vi "FinalLabview.vi"() -> ()   [LabVIEW 2021]
panel:
  out "DummyIndicator 5":dbl
  out "Ball Color":dbl
  out "DummyIndicator 3":dbl
  out "Ball Count":dbl
  out "Ball Color 5":string
  out "Ball Color 4":string
  out "Ball Color 3":string
  out "Ball Color 2":string
  out "Ball Color 1":string
  out "Y Coordinate 5":dbl
  out "X Coordinate 5":dbl
  out "Y Coordinate 4":dbl
  out "X Coordinate 4":dbl
  out "Y Coordinate 3":dbl
  out "X Coordinate 3":dbl
  out "Y Coordinate 2":dbl
  out "X Coordinate 2":dbl
  out "2D Picture":picture
  in  "Display History":bool
  in  "Size of Rectangle":i16
  out "Y Coordinate 1":dbl
  out "X Coordinate 1":dbl
  out "Y":dbl
  out "X":dbl
  in  "SendValue8":dbl
  in  "SendValue7":dbl
  in  "SendValue6":dbl
  in  "SendValue5":dbl
  in  "SendValue4":dbl
  in  "SendValue3":dbl
  in  "SendValue2":dbl
  in  "SendValue1":dbl
  in  "Send Button":bool
  in  "Stop Button":bool
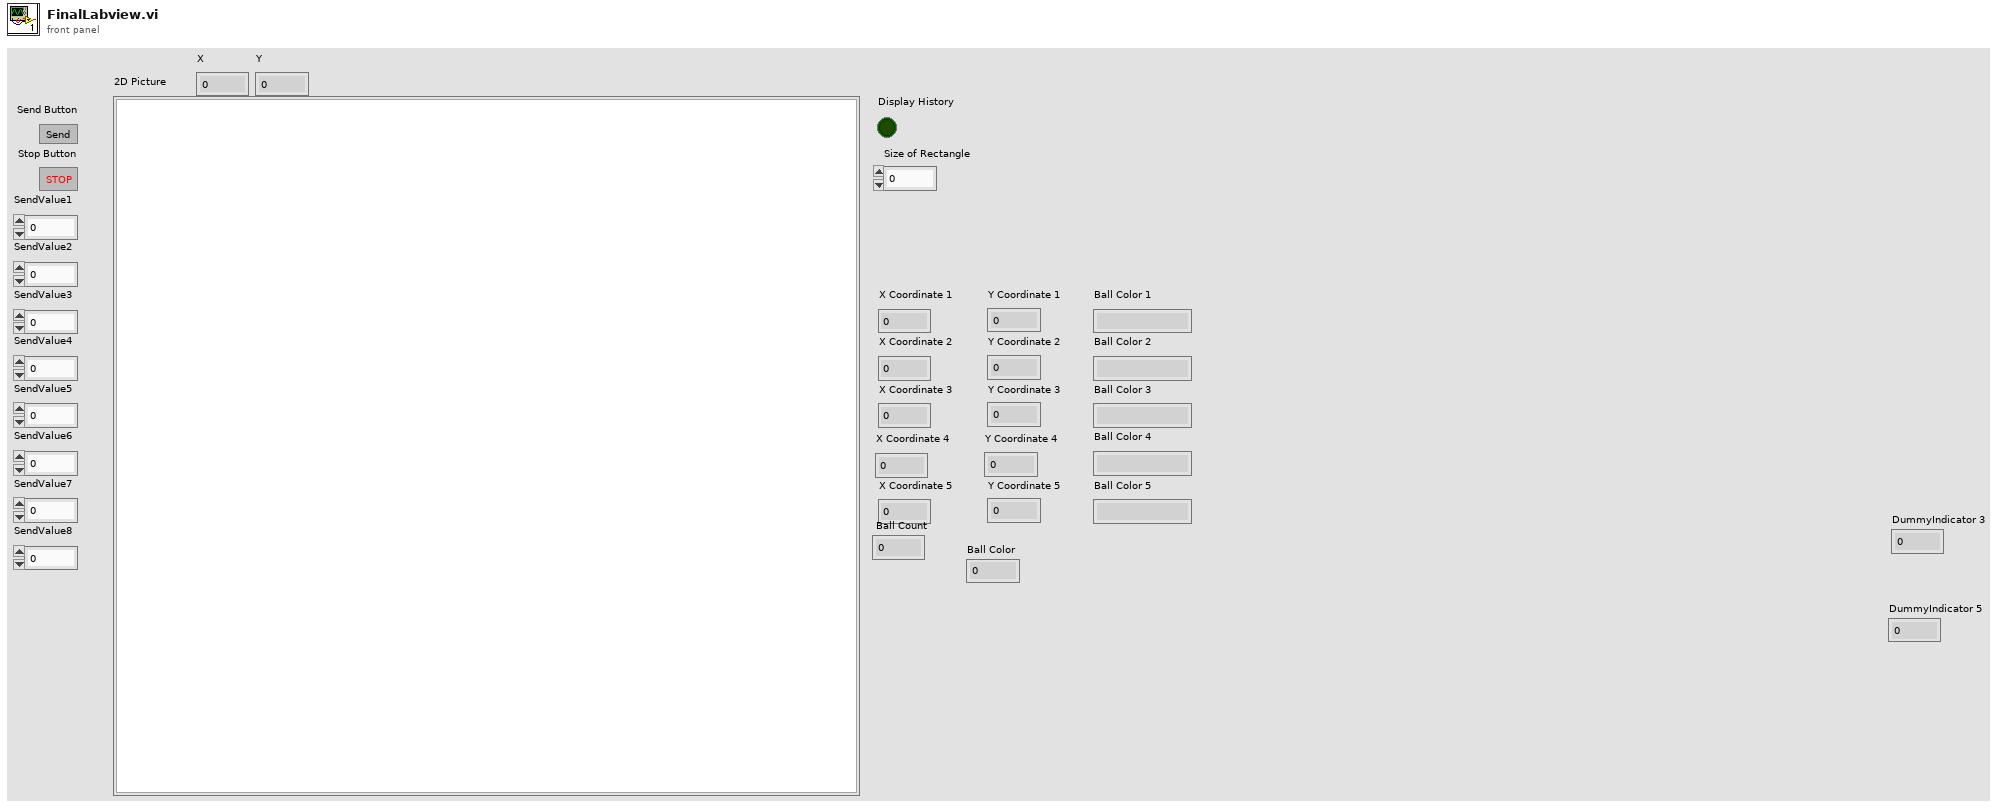
[diagram p1: front panel]
types:
  T1 = cluster{"Width":u16, "Style":enum32{"Solid", "Dash", "Dot", "DashDot", "DashDotDot"}}
  T2 = cluster{"Width":i16, "Style":enum32{"Solid", "Dash", "Dot", "DashDot", "DashDotDot"}}
  T3 = cluster{"left":i16, "top":i16, "right":i16, "bottom":i16}
  T4 = enum16{"Standard", "Buffered", "CRLF", "Immediate"}
  T5 = cluster{"default value 1":dbl, "default value 1":dbl}
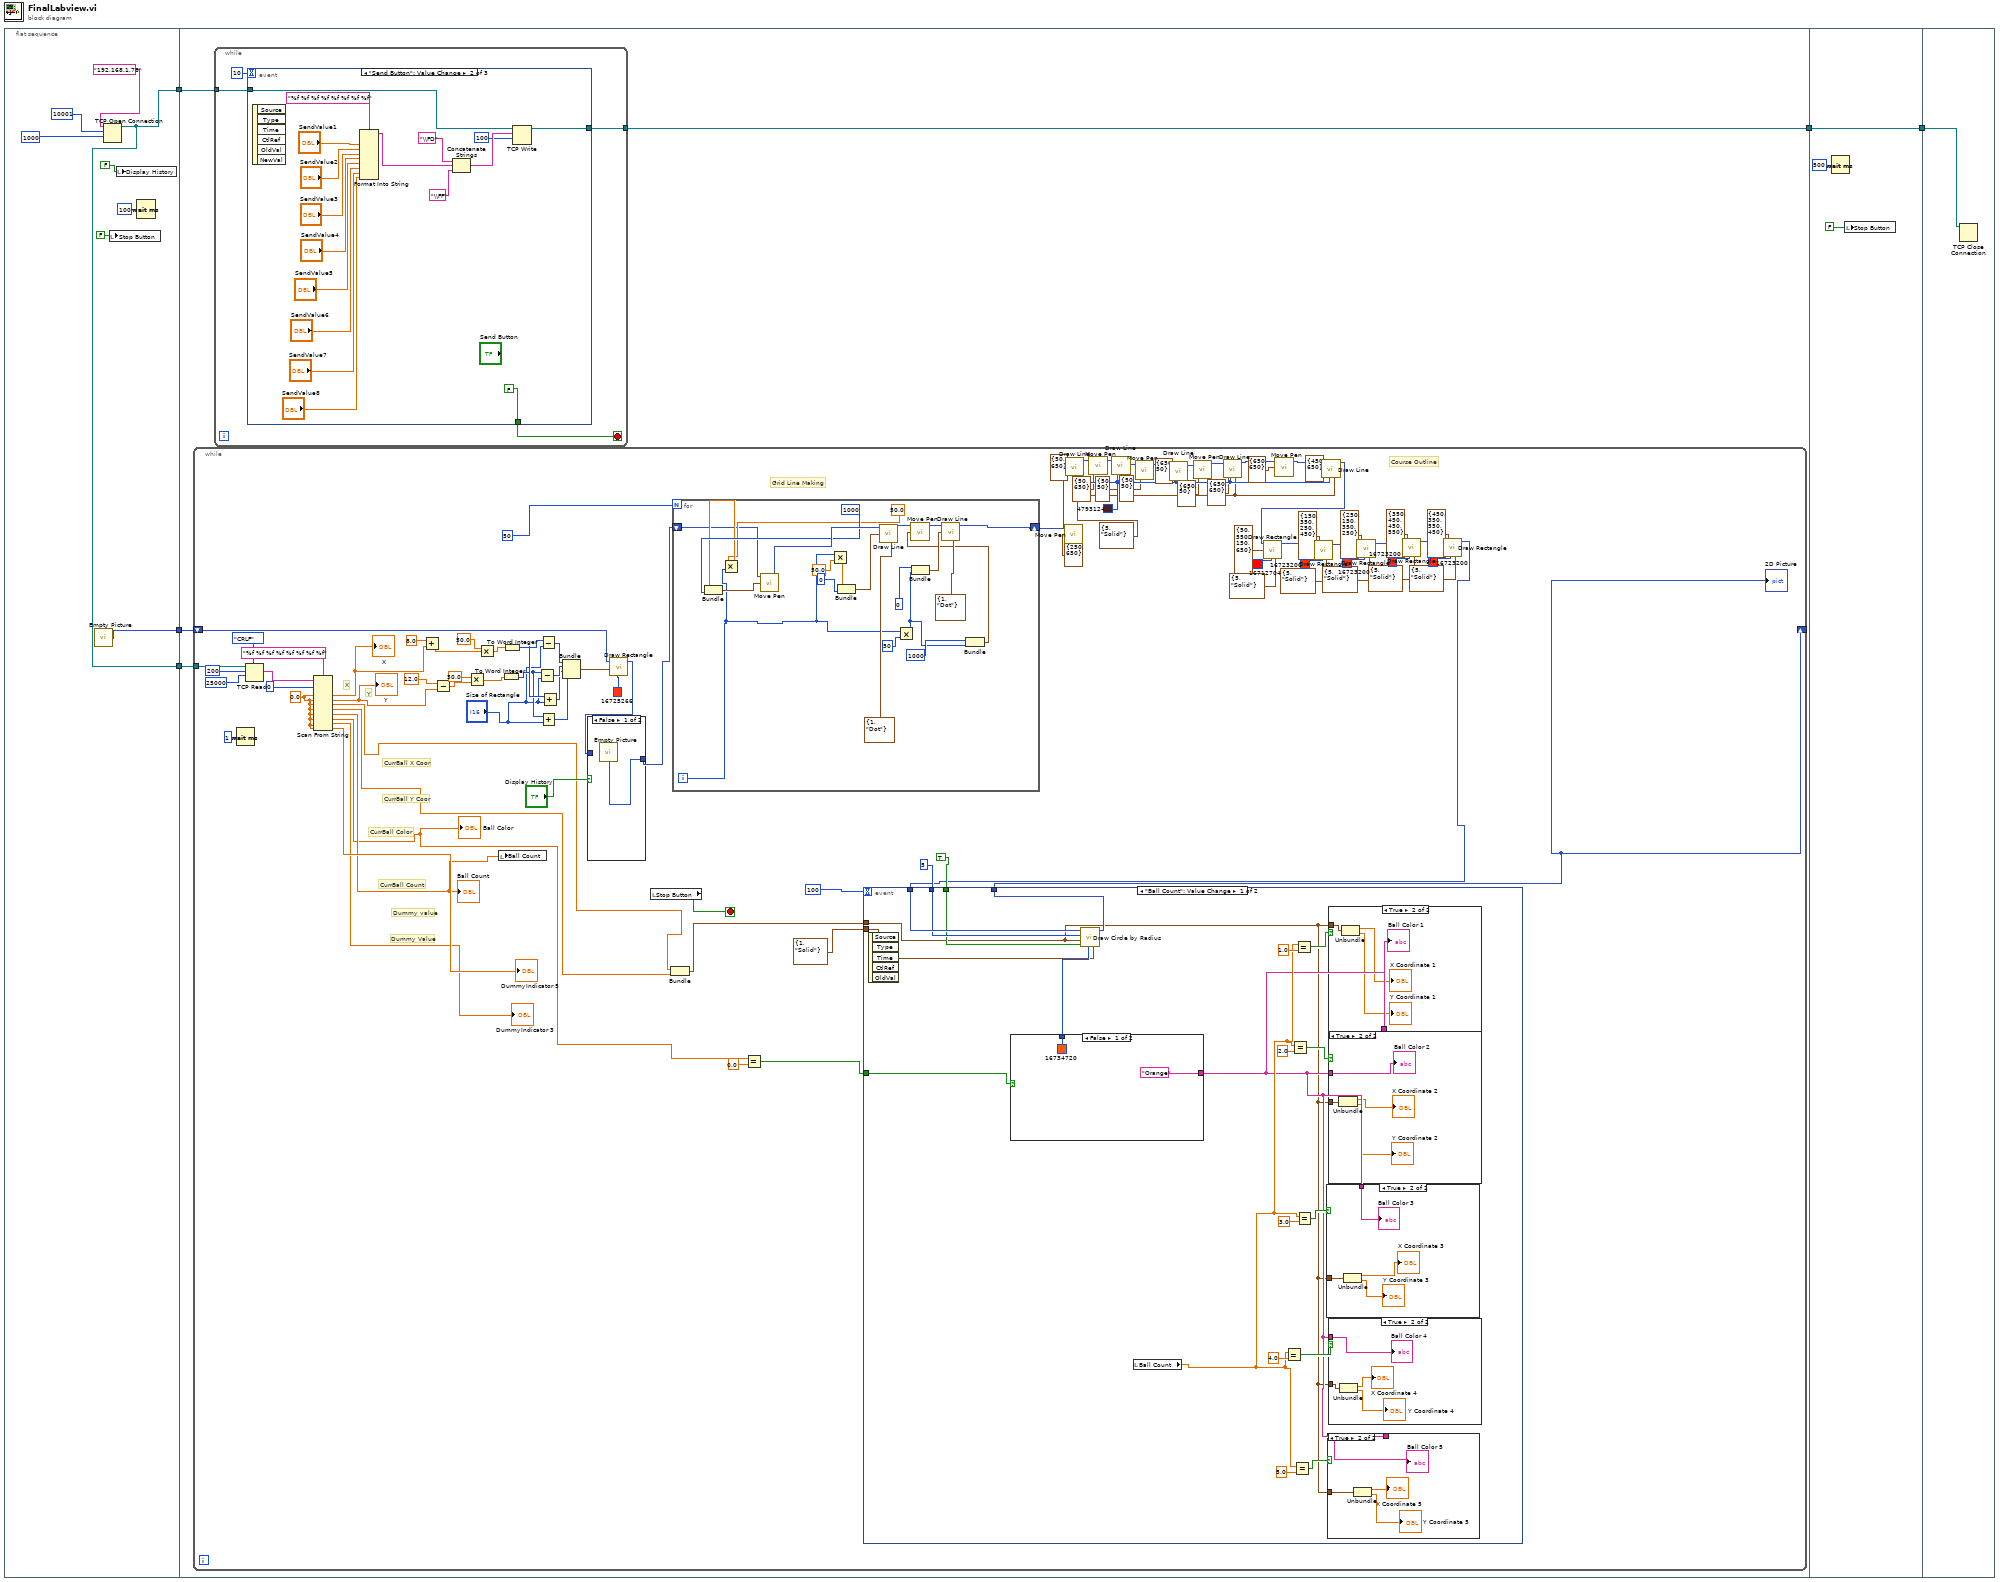
[diagram p0: block diagram]
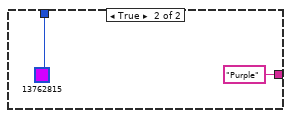
[diagram p7: hidden frame]
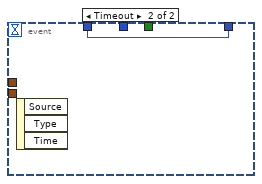
[diagram p8: hidden frame]
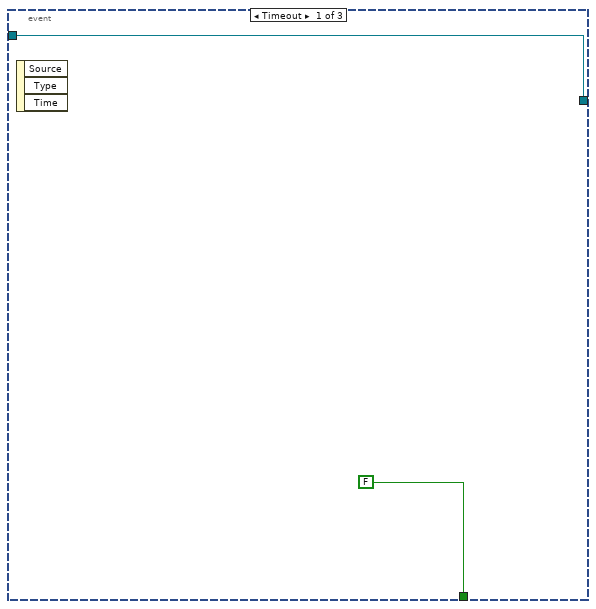
[diagram p10: hidden frame]
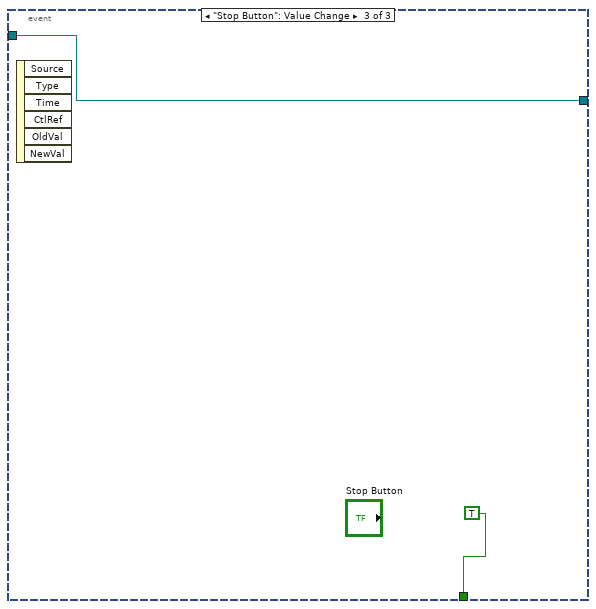
[diagram p11: hidden frame]
diagram:
  n1 = flat-sequence {
    tunnel: [w6] -> w5
    tunnel: [w8] -> w2
    tunnel: [w6] -> w1
    tunnel: w5 -> [w17]
    tunnel: [w16] -> w3
    tunnel: w2 -> [w14]
    tunnel: w1 -> [w15]
    tunnel: [w203] -> w4
    tunnel: w3 -> [w203]
    tunnel: w4 -> [w206]
    frame #0 {
      n2 = call "Empty Picture"() -> ("empty picture"=w8:picture)
      n3 = TCP Open Connection(address="192.168.1.78", remote port or service name=u16 10001, timeout ms (60000)=1000) -> (connection ID=w6:refnum<k5>)  [unwired: 2 in, 1 out]
      n4 = local write "Stop Button"(FALSE) -> ()
      n5 = local write "Display History"(FALSE) -> ()
      n6 = Wait (ms)(milliseconds to wait=u32 100) -> ()  [unwired: 1 out]
    }
    frame #1 {
      n7 = while {
        tunnel: w15 -> [w107]
        shift-right: [w18] -> _
        shift-left: w14 -> [w83]
        stop <- w80 stop-if-true
        w51 = T1 {"Width"=5, "Style"=enum."Solid"} ("pen")
        w52 = u32 4793124 ("color(black)")
        w32 = 0.0 ("default value 1")
        # "Dummy Value"
        # "CurrBall Count"
        # "Dummy value"
        # "CurrBall Color"
        # "CurrBall Y Coor"
        # "CurrBall X Coor"
        # "Y"
        # "X"
        # "Course Outline"
        # "Grid Line Making"
        n8 = Wait (ms)(milliseconds to wait=u32 1) -> ()  [unwired: 1 out]
        n9 = TCP Read(connection ID=w107, bytes to read=200, 7:T4."CRLF" ("mode (standard)"), 9:25000 ("timeout ms (25000)")) -> (data out=w103:string)  [unwired: 1 in, 2 out]
        n10 = Scan From String(format string="%f %f %f %f %f %f %f %f", input string=w103, initial scan location=u32 0, default 1=w32, default 2=w32, default 3=w32, default 4=w32, default 5=w32, default 6=w32, default 7=w32, default 8=w32) -> (output 1=w100:dbl, output 2=w31:dbl, output 3=w54:dbl, output 4=w28:dbl, output 5=w24:dbl, output 6=w23:dbl, output 7=→"DummyIndicator 3":dbl, output 8=→"DummyIndicator 5":dbl)  [unwired: 1 in, 3 out]
        "X" <- w100
        "Y" <- w31
        "Ball Count" <- w24
        "Ball Color" <- w23
        n11 = Add(x=8.0, y=w100) -> (x+y=w97:dbl)
        n12 = Subtract(x=12.0, y=w31) -> (x-y=w95:dbl)
        n13 = Multiply(x=50.0, y=w95) -> (x*y=w92:dbl)
        n14 = Multiply(x=50.0, y=w97) -> (x*y=w93:dbl)
        n15 = local write "Ball Count"(w24) -> ()
        n16 = To Word Integer(number=w92) -> (16bit integer=w90:i16)
        n17 = To Word Integer(number=w93) -> (16bit integer=w91:i16)
        n18 = Subtract(x=w90, y="Size of Rectangle") -> (x-y=w87:i16)
        n19 = Subtract(x=w91, y="Size of Rectangle") -> (x-y=w88:i16)
        n20 = Add(x=w90, y="Size of Rectangle") -> (x+y=w85:i16)
        n21 = Add(x=w91, y="Size of Rectangle") -> (x+y=w86:i16)
        n22 = Bundle(w88, w87, w86, w85) -> (w82:cluster{i16, i16, i16, i16})  [unwired: 1 in]
        n23 = call <vilib>:"Draw Rectangle.vi"("picture"=w83, "rect"=w82, "color(black)"=u32 16725266) -> ("new picture"=w22:picture)  [unwired: 6 in]
        n24 = case shown="False" "Display History" {
          tunnel: w22 -> [_ w177]
          tunnel: [w176 w177] -> w21
          frame False {
            n25 = call "Empty Picture"() -> ("empty picture"=w176:picture)
          }
          frame True {
          }
        }
        n26 = local read "Stop Button"() -> (w80:bool)
        n27 = Bundle("default value 1"=w54, "default value 1"=w28) -> (w27:T5)  [unwired: 1 in]
        n28 = for {
          N: 50 -> [_]
          shift-right: [w170] -> w77
          shift-left: w21 -> [w154]
          i -> [w155]
          n29 = Multiply(x=50.0, y=w155) -> (x*y=w160:dbl)
          n30 = Bundle(w160, 1000) -> (w162:cluster{dbl, i32})  [unwired: 1 in]
          n31 = call <vilib>:"Move Pen.vi"("new position"=w162, "picture"=w154) -> ("new picture"=w166:picture)  [unwired: 3 in]
          n32 = Multiply(x=w155, y=50.0) -> (x*y=w174:dbl)
          n33 = Bundle(w174, 0) -> (w172:cluster{dbl, i32})  [unwired: 1 in]
          n34 = call <vilib>:"Draw Line.vi"("picture"=w166, "end point"=w172, "pen"=T1 {"Width"=1, "Style"=enum."Dot"}) -> ("new picture"=w164:picture)  [unwired: 6 in]
          n35 = Multiply(x=w155, y=50) -> (x*y=w156:i32)
          n36 = Bundle(0, w156) -> (w168:cluster{i32, i32})  [unwired: 1 in]
          n37 = Bundle(1000, w156) -> (w158:cluster{i32, i32})  [unwired: 1 in]
          n38 = call <vilib>:"Move Pen.vi"("new position"=w158, "picture"=w164) -> ("new picture"=w165:picture)  [unwired: 3 in]
          n39 = call <vilib>:"Draw Line.vi"("picture"=w165, "end point"=w168, "pen"=T1 {"Width"=1, "Style"=enum."Dot"}) -> ("new picture"=w170:picture)  [unwired: 6 in]
        }
        n40 = Equal?(x=w23, y=0.0) -> (x = y?=w29:bool)
        n41 = call <vilib>:"Move Pen.vi"("new position"=cluster{"x":i16, "y":i16} {"x"=250, "y"=650}, "picture"=w77) -> ("new picture"=w53:picture)  [unwired: 3 in]
        n42 = call <vilib>:"Draw Line.vi"("picture"=w53, "end point"=cluster{"x":i16, "y":i16} {"x"=50, "y"=650}, "color(black)"=w52, "pen"=w51) -> ("new picture"=w49:picture)  [unwired: 5 in]
        n43 = call <vilib>:"Move Pen.vi"("new position"=cluster{"x":i16, "y":i16} {"x"=50, "y"=650}, "picture"=w49) -> ("new picture"=w48:picture)  [unwired: 3 in]
        n44 = call <vilib>:"Draw Line.vi"("picture"=w48, "end point"=cluster{"x":i16, "y":i16} {"x"=50, "y"=50}, "color(black)"=w52, "pen"=w51) -> ("new picture"=w41:picture)  [unwired: 5 in]
        n45 = call <vilib>:"Move Pen.vi"("new position"=cluster{"x":i16, "y":i16} {"x"=50, "y"=50}, "picture"=w41) -> ("new picture"=w40:picture)  [unwired: 3 in]
        n46 = call <vilib>:"Draw Line.vi"("picture"=w40, "end point"=cluster{"x":i16, "y":i16} {"x"=650, "y"=50}, "color(black)"=w52, "pen"=w51) -> ("new picture"=w42:picture)  [unwired: 5 in]
        n47 = call <vilib>:"Move Pen.vi"("new position"=cluster{"x":i16, "y":i16} {"x"=650, "y"=50}, "picture"=w42) -> ("new picture"=w45:picture)  [unwired: 3 in]
        n48 = call <vilib>:"Draw Line.vi"("picture"=w45, "end point"=cluster{"x":i16, "y":i16} {"x"=650, "y"=650}, "color(black)"=w52, "pen"=w51) -> ("new picture"=w43:picture)  [unwired: 5 in]
        n49 = call <vilib>:"Move Pen.vi"("new position"=cluster{"x":i16, "y":i16} {"x"=650, "y"=650}, "picture"=w43) -> ("new picture"=w44:picture)  [unwired: 3 in]
        n50 = call <vilib>:"Draw Line.vi"("picture"=w44, "end point"=cluster{"x":i16, "y":i16} {"x"=450, "y"=650}, "color(black)"=w52, "pen"=w51) -> ("new picture"=w47:picture)  [unwired: 5 in]
        n51 = call <vilib>:"Draw Rectangle.vi"("picture"=w47, "rect"=T3 {"left"=50, "top"=550, "right"=150, "bottom"=650}, "color(black)"=u32 16712704, "pen"=T2 {"Width"=5, "Style"=enum."Solid"}) -> ("new picture"=w73:picture)  [unwired: 5 in]
        n52 = call <vilib>:"Draw Rectangle.vi"("picture"=w73, "rect"=T3 {"left"=150, "top"=350, "right"=250, "bottom"=450}, "color(black)"=u32 16723200, "pen"=T2 {"Width"=5, "Style"=enum."Solid"}) -> ("new picture"=w72:picture)  [unwired: 5 in]
        n53 = call <vilib>:"Draw Rectangle.vi"("picture"=w72, "rect"=T3 {"left"=250, "top"=150, "right"=350, "bottom"=250}, "color(black)"=u32 16723200, "pen"=T2 {"Width"=5, "Style"=enum."Solid"}) -> ("new picture"=w71:picture)  [unwired: 5 in]
        n54 = call <vilib>:"Draw Rectangle.vi"("picture"=w71, "rect"=T3 {"left"=350, "top"=450, "right"=450, "bottom"=550}, "color(black)"=u32 16723200, "pen"=T2 {"Width"=5, "Style"=enum."Solid"}) -> ("new picture"=w70:picture)  [unwired: 5 in]
        n55 = call <vilib>:"Draw Rectangle.vi"("picture"=w70, "rect"=T3 {"left"=450, "top"=350, "right"=550, "bottom"=450}, "color(black)"=u32 16723200, "pen"=T2 {"Width"=5, "Style"=enum."Solid"}) -> ("new picture"=w19:picture)  [unwired: 5 in]
        n56 = event shown="[0] \"Ball Count\": Value Change" {
          selector: _ -> [_ _]
          dyn-events: _ -> [_ _]
          timeout: 100 -> [_ _]
          tunnel: [w128 w153] -> w18
          tunnel: w19 -> [w127 w153]
          tunnel: i16 5 ("radius") -> [w125 _]
          tunnel: TRUE ("fill?(F)") -> [w124 _]
          tunnel: T1 {"Width"=1, "Style"=enum."Solid"} ("pen") -> [w123 _]
          tunnel: w29 -> [w122 _]
          tunnel: w27 -> [w109 _]
          event "Ball Count": Value Change {
            n57 = event-data() -> ()  [unwired: 1 in, 5 out]
            n58 = case shown="False" w122 {
              tunnel: [u32 16734720 ("color(black)") u32 13762815 ("color(black)")] -> w126
              tunnel: ["Orange" ("Ball Color 1") "Purple" ("Ball Color 1")] -> w110
              frame False {
              }
              frame True {
              }
            }
            n59 = call <vilib>:"Draw Circle by Radius.vi"("pen"=w123, "color(black)"=w126, "fill?(F)"=w124, "pixel center"=w109, "radius"=w125, "picture"=w127) -> ("new picture"=w128:picture)  [unwired: 5 in]
            n60 = local read "Ball Count"() -> (w112:dbl)
            n61 = Equal?(x=w112, y=4.0) -> (x = y?=w115:bool)
            n62 = Equal?(x=w112, y=2.0) -> (x = y?=w111:bool)
            n63 = Equal?(x=w112, y=5.0) -> (x = y?=w114:bool)
            n64 = Equal?(x=w112, y=1.0) -> (x = y?=w121:bool)
            n65 = Equal?(x=w112, y=3.0) -> (x = y?=w113:bool)
            n66 = case shown="True" w113 {
              tunnel: w110 -> [_ w140]
              tunnel: w109 -> [_ w139]
              frame False {
              }
              frame True {
                n67 = Unbundle(w139) -> ("default value 1"=→"X Coordinate 3":dbl, "default value 1"=→"Y Coordinate 3":dbl)
                "Ball Color 3" <- w140
              }
            }
            n68 = case shown="True" w114 {
              tunnel: w110 -> [_ w132]
              tunnel: w109 -> [_ w131]
              frame False {
              }
              frame True {
                n69 = Unbundle(w131) -> ("default value 1"=→"X Coordinate 5":dbl, "default value 1"=→"Y Coordinate 5":dbl)
                "Ball Color 5" <- w132
              }
            }
            n70 = case shown="True" w111 {
              tunnel: w110 -> [_ w144]
              tunnel: w109 -> [_ w143]
              frame False {
              }
              frame True {
                n71 = Unbundle(w143) -> ("default value 1"=→"X Coordinate 2":dbl, "default value 1"=→"Y Coordinate 2":dbl)
                "Ball Color 2" <- w144
              }
            }
            n72 = case shown="True" w115 {
              tunnel: w110 -> [_ w136]
              tunnel: w109 -> [_ w135]
              frame False {
              }
              frame True {
                n73 = Unbundle(w135) -> ("default value 1"=→"X Coordinate 4":dbl, "default value 1"=→"Y Coordinate 4":dbl)
                "Ball Color 4" <- w136
              }
            }
            n74 = case shown="True" w121 {
              tunnel: w109 -> [_ w148]
              tunnel: w110 -> [_ w147]
              frame False {
              }
              frame True {
                n75 = Unbundle(w148) -> ("default value 1"=→"X Coordinate 1":dbl, "default value 1"=→"Y Coordinate 1":dbl)
                "Ball Color 1" <- w147
              }
            }
          }
          event Timeout {
            n76 = event-data() -> ()  [unwired: 1 in, 3 out]
          }
        }
        "2D Picture" <- w18
      }
      n77 = while {
        tunnel: w17 -> [w179]
        tunnel: [w178] -> w16
        stop <- w180 stop-if-true
        n78 = event shown="[1] \"Send Button\": Value Change" {
          selector: _ -> [_ _ _]
          dyn-events: _ -> [_ _ _]
          timeout: 10 -> [_ _ _]
          tunnel: [FALSE FALSE TRUE] -> w180
          tunnel: w179 -> [w182 w185 w201]
          tunnel: [w182 w184 w201] -> w178
          event Timeout {
            n79 = event-data() -> ()  [unwired: 1 in, 3 out]
          }
          event "Send Button": Value Change {
            n80 = event-data() -> ()  [unwired: 1 in, 6 out]
            n81 = Format Into String(format string="%f %f %f %f %f %f %f %f", "SendValue1", "SendValue2", "SendValue3", "SendValue4", "SendValue5", "SendValue6", "SendValue7", "SendValue8") -> (resulting string=w187:string)  [unwired: 2 in, 1 out]
            n82 = Concatenate Strings("\\FD" ("string"), w187, "\\FF" ("string")) -> (w190:string)
            n83 = TCP Write(connection ID=w185, data in=w190, 9:100 ("timeout ms (25000)")) -> (connection ID out=w184:refnum<k5>)  [unwired: 1 in, 2 out]
          }
          event "Stop Button": Value Change {
            n84 = event-data() -> ()  [unwired: 1 in, 6 out]
          }
        }
      }
    }
    frame #2 {
      n85 = Wait (ms)(milliseconds to wait=u32 500) -> ()  [unwired: 1 out]
      n86 = local write "Stop Button"(FALSE) -> ()
    }
    frame #3 {
      n87 = TCP Close Connection(connection ID=w206) -> ()  [unwired: 2 in, 2 out]
    }
  }
